vi "talk_to_observers2.vi"(7 "force sending?":bool=TRUE, 8 "error in (no error)":errorcluster, 9 "image finished?":bool=TRUE, 10 "image (channels)":refnum<class "Image.lvclass">[](array[class]), 11 "GenericToplevelComponent in":refnum<class "GenericToplevelComponent.lvclass">) -> (0 "error out":errorcluster, 3 "GenericToplevelComponent out":refnum<class "GenericToplevelComponent.lvclass">)   [LabVIEW 2010, in "GenericToplevelComponent.lvclass"]
uses:
  GenericToplevelComponent.lvclass
  Image/Image/Image.lvclass
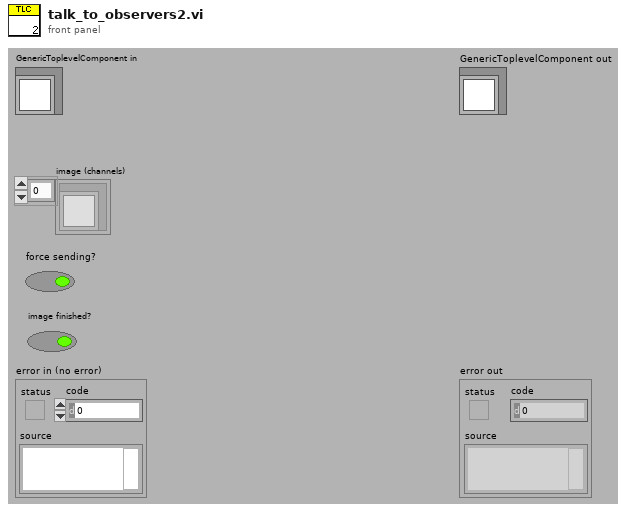
[diagram p1: front panel]
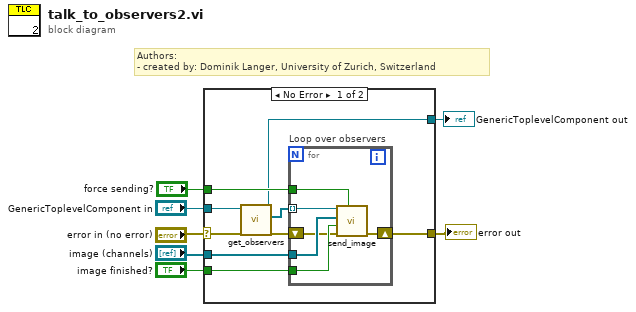
[diagram p0: block diagram]
diagram:
  # "Authors: \n- created by: Dominik Langer, University of Zurich, Switzerland"
  n1 = case shown="No Error" "error in (no error)" {
    selector: "error in (no error)" -> [w9 w24]
    tunnel: [w16 w24] -> w4
    tunnel: [w11 w23] -> w3
    tunnel: "GenericToplevelComponent in" -> [w12 w23]
    tunnel: "image (channels)" -> [w15 _]
    tunnel: "image finished?" -> [w14 _]
    tunnel: "force sending?" -> [w13 _]
    frame No Error {
      n2 = call-dynamic "get_observers.vi"("error in (no error)"=w9, "GenericToplevelComponent in"=w12) -> ("error out"=w8:errorcluster, "observers"=w10:refnum<class "GenericToplevelComponent.lvclass">[], "GenericToplevelComponent out"=w11:refnum<class "GenericToplevelComponent.lvclass">)  [unwired: 7 in]
      n3 = for "Loop over observers" {
        shift-right: [w22] -> w16
        shift-left: w8 -> [w18]
        tunnel: w15 -> [w21]
        tunnel: w14 -> [w20]
        tunnel: w13 -> [w19]
        tunnel: w10 -> [w17] mode=indexing
        n4 = call-dynamic "send_image.vi"("force sending?"=w19, "error in (no error)"=w18, "image finished?"=w20, "image (channels)"=w21, "GenericToplevelComponent in"=w17) -> ("error out"=w22:errorcluster)  [unwired: 4 in, 2 out]
      }
    }
    frame Error {
    }
  }
  "error out" <- w4
  "GenericToplevelComponent out" <- w3
